vi "TwoBallAuto2safeHangar.vi"() -> ()   [LabVIEW 2020]
uses:
  Global Variables/AutoOneBall.ctl
  <vilib>/Rock Robotics/WPI/ThirdParty/REV Robotics/REVLib/Typedef/Spark MAX Control Type.ctl
  Global Variables/ActuatorsSensors.vi
  Global Variables/Axes_N_Buttons.vi
panel:
  in  "Tab Control":T1(tab)
  out "R Output":cluster{"Applied Output":dbl}(graph)
  out "L Output":cluster{"Applied Output":dbl}(graph)
  out "PID R":cluster{"Sensor Position":dbl, "Setpoint":dbl}(graph)
  out "PID L":cluster{"Sensor Position":dbl, "Setpoint":dbl}(graph)
  in  "Reset":bool
  in  "PID Constants L":T2={"P Gain"=0.007, "I Gain"=0.0002, "D Gain"=0.0, "F Gain"=0.0, "I Zone"=1000.0, "Min Output"=-1.0, "Max Output"=1.0}
  in  "PID Constants R":T2={"P Gain"=0.003, "I Gain"=0.0002, "D Gain"=0.0, "F Gain"=0.0, "I Zone"=1000.0, "Min Output"=-0.1, "Max Output"=0.1}
  in  "Range":cluster{"output high":dbl, "output low":dbl}={"output high"=0.6, "output low"=-0.6} {"output low" format="%.2f"; "output high" format="%.2f"}
  in  "Gains":T3={"proportional gain (Kc)"=0.04, "integral time (Ti, min)"=0.0, "derivative time (Td, min)"=0.0} {"derivative time (Td, min)" format="%.3f"; "integral time (Ti, min)" format="%.3f"; "proportional gain (Kc)" format="%.3f"}
  in  "Soft start":dbl=1.8 format="%#_13g"
  in  "Meters":dbl=-2.5
  in  "Meters 2":dbl=2.3
  in  "Range 2":cluster{"output high":dbl, "output low":dbl}={"output high"=0.45, "output low"=-0.45} {"output low" format="%.2f"; "output high" format="%.2f"}
  in  "Meters 3":dbl=-0.6
  in  "Meters 4":dbl=-0.6
  in  "Meters 5":dbl=-1.5
  in  "Meters 6":dbl=-1.0
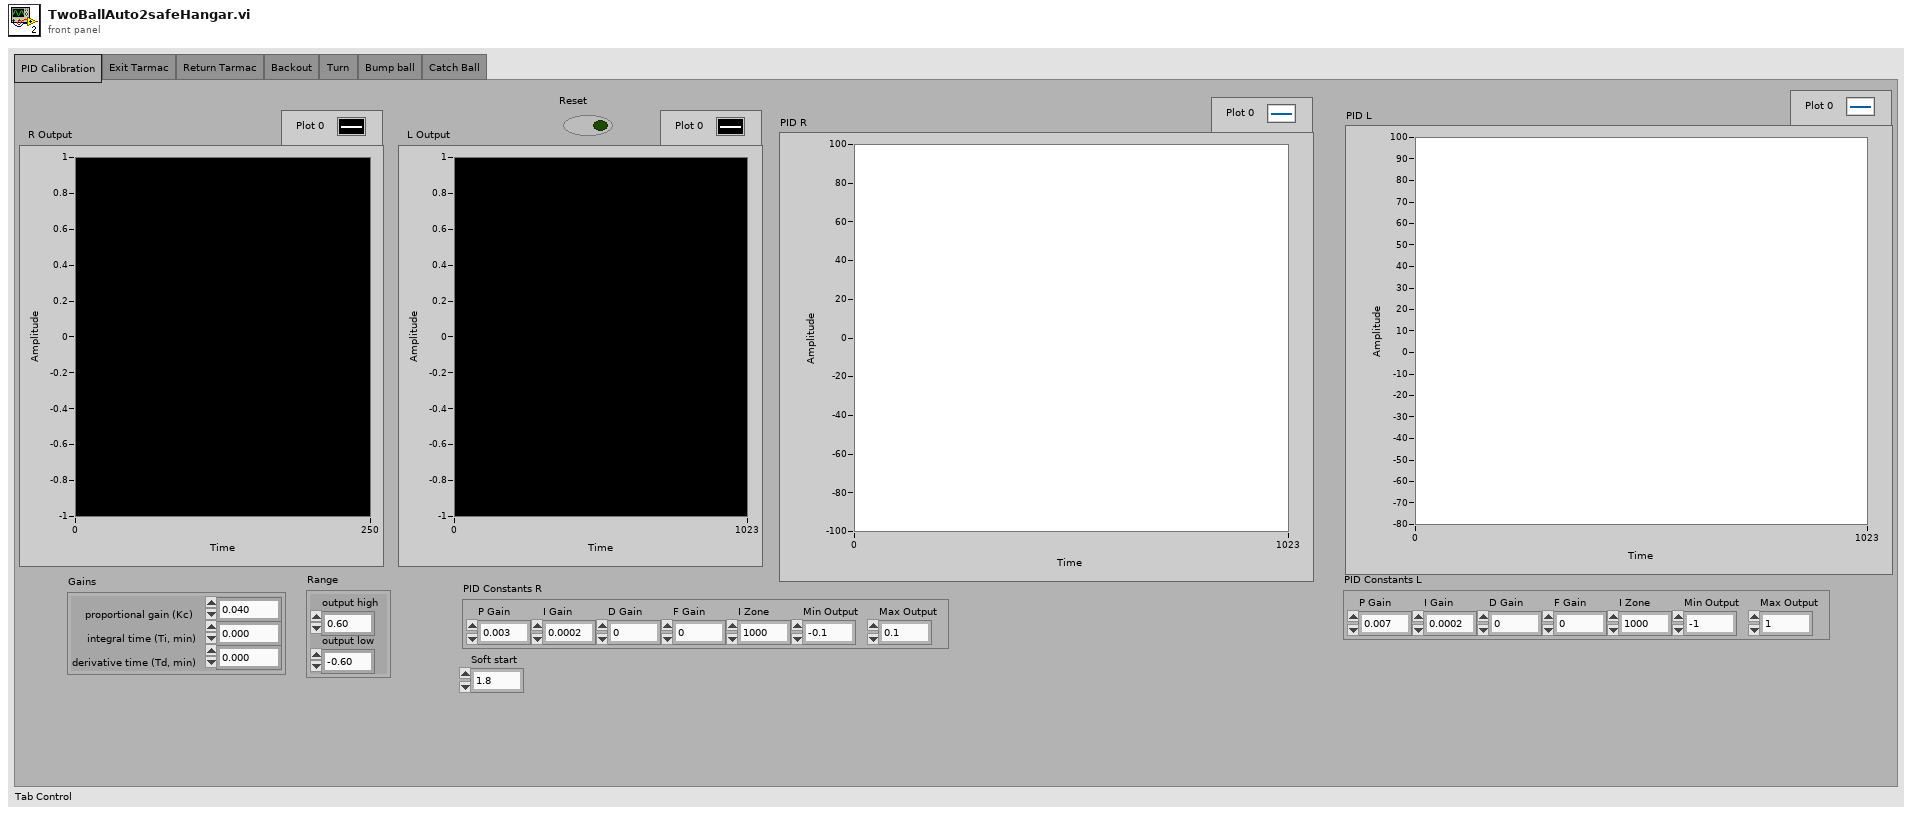
[diagram p1: front panel]
types:
  T1 = enum32{"PID Calibration", "Exit Tarmac", "Return Tarmac", "Backout", "Turn ", "Bump ball", "Catch Ball"}
  T2 = cluster{"P Gain":dbl, "I Gain":dbl, "D Gain":dbl, "F Gain":dbl, "I Zone":dbl, "Min Output":dbl, "Max Output":dbl}
  T3 = cluster{"proportional gain (Kc)":dbl, "integral time (Ti, min)":dbl, "derivative time (Td, min)":dbl}
  T4 = typedef "AutoOneBall.ctl" = enum16{"Start", "Shoot", "Delay", "Exit Tarmac", "Delay 2", "Return Tarmac", "Delay 3", "Prepare Shooter 2", "Align", "Shoot 2", "Backout", "Delay 4", "Turn", "Delay 5", "Bump Ball", "Collect Ball", "Reset"}
  T5 = typedef "WPI_MotorControlDeviceRef.ctl" = cluster{"DeviceStatus":errorcluster, "Type":T6, "PWM":cluster{"PWM Channel":T7, "DeadBand":T8}, "CAN":cluster{"Device Number":u8, "SetOutput VI Ref":variant, "GetOutput VI Ref":variant, "Enable VI Ref":variant, "Disable VI Ref":variant, "Data":variant}, "Invert":bool, "DIO PWM":cluster{"PWM \"Enable\" Channel":T7, "DIOChannel":T9, "PWM Rate":dbl}}
  T6 = typedef "WPI_MotorControlType.ctl" = enum16{"PWM", "CAN", "DIO PWM"}
  T7 = typedef "FPGA_DIOPWMChannel.ctl" = enum8{"PWM 0", "PWM 1", "PWM 2", "PWM 3", "PWM 4", "PWM 5", "PWM 6", "PWM 7", "PWM 8", "PWM 9", "PWM MXP 0", "PWM MXP 1", "PWM MXP 2", "PWM MXP 3", "PWM MXP 4", "PWM MXP 5", "PWM MXP 6", "PWM MXP 7", "PWM MXP 8", "PWM MXP 9", "Invalid"}
  T8 = typedef "WPI_PWMDeadband.ctl" = cluster{"Name":string, "maxPositivePwm":i32, "minPositivePwm":i32, "centerPwm":i32, "maxNegativePwm":i32, "minNegativePwm":i32, "angularRange":u16}
  T9 = typedef "FPGA_DIOChannel.ctl" = enum8{"DIO 0", "DIO 1", "DIO 2", "DIO 3", "DIO 4", "DIO 5", "DIO 6", "DIO 7", "DIO 8", "DIO 9", "DIO MXP 0", "DIO MXP 1", "DIO MXP 2", "DIO MXP 3", "DIO MXP 4", "DIO MXP 5", "DIO MXP 6", "DIO MXP 7", "DIO MXP 8", "DIO MXP 9", "DIO MXP 10", "DIO MXP 11", "DIO MXP 12", "DIO MXP 13", "DIO MXP 14", "DIO MXP 15", "SPI Port CS1", "SPI Port CS2", "SPI Port CS3", "SPI Port MISO", "SPI Port MOSI", "Invalid"}
  T10 = typedef "Spark MAX Control Type.ctl" = enum16{"Percent VBus", "Voltage", "Velocity", "Position", "Smart Motion", "Current", "Smart Velocity"}
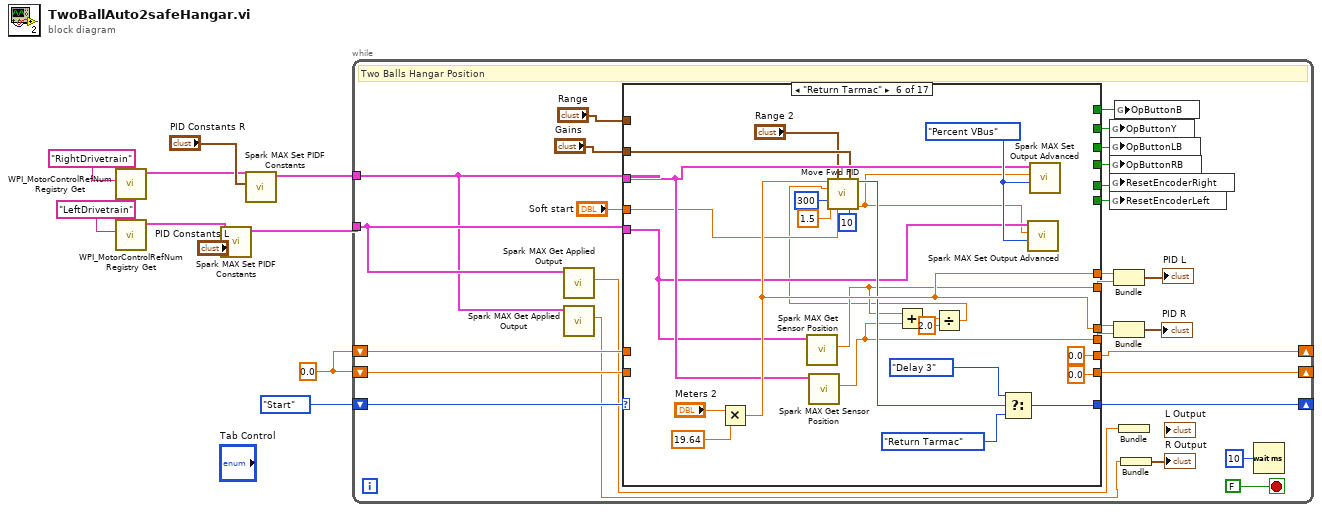
[diagram p0: block diagram]
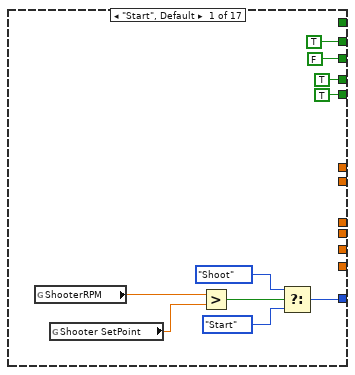
[diagram p2: hidden frame]
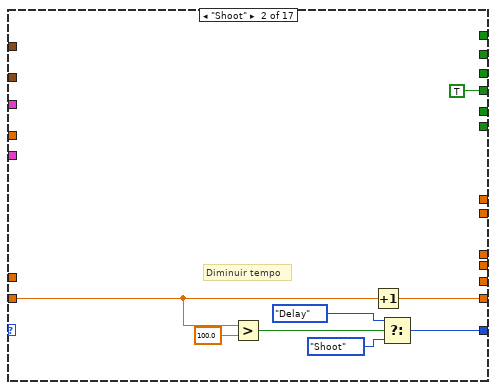
[diagram p3: hidden frame]
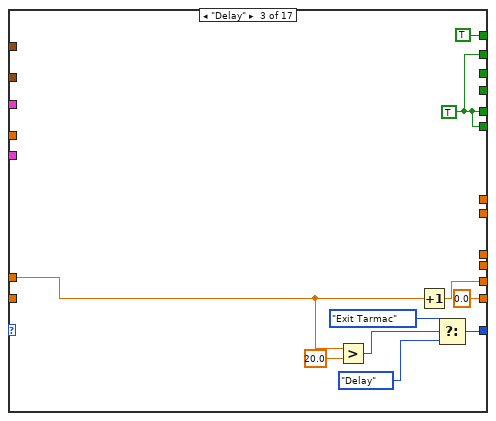
[diagram p4: hidden frame]
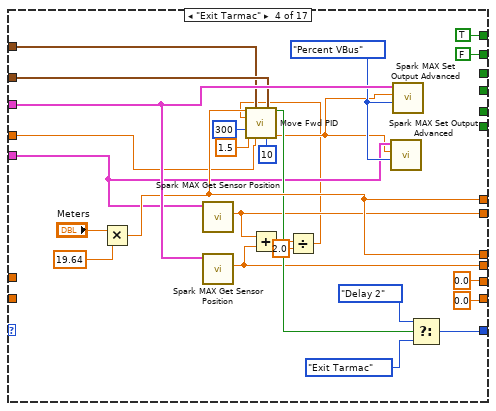
[diagram p5: hidden frame]
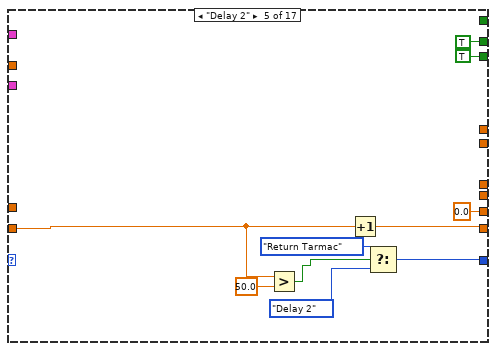
[diagram p6: hidden frame]
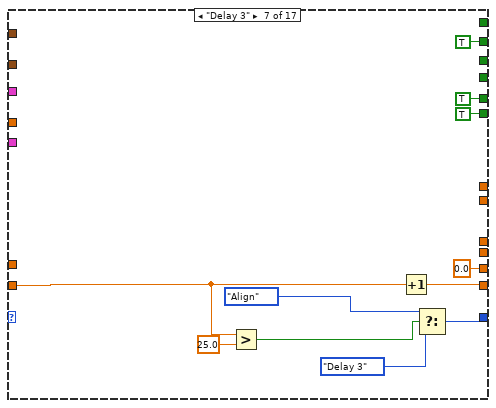
[diagram p7: hidden frame]
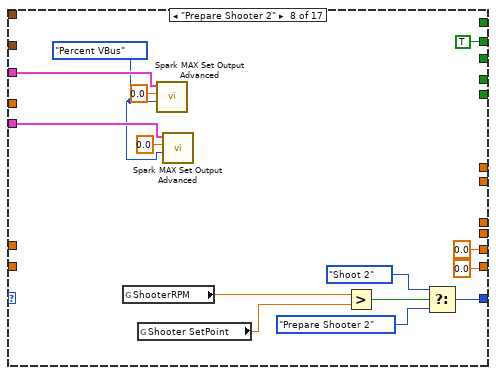
[diagram p8: hidden frame]
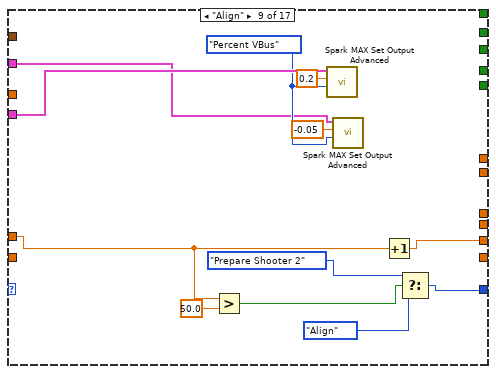
[diagram p9: hidden frame]
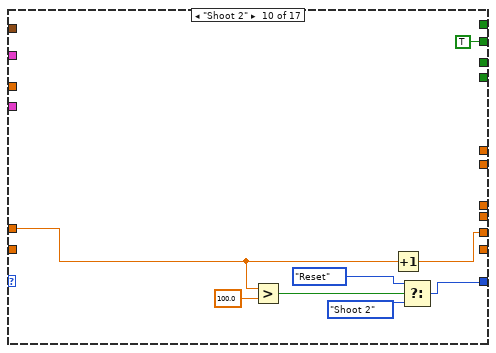
[diagram p10: hidden frame]
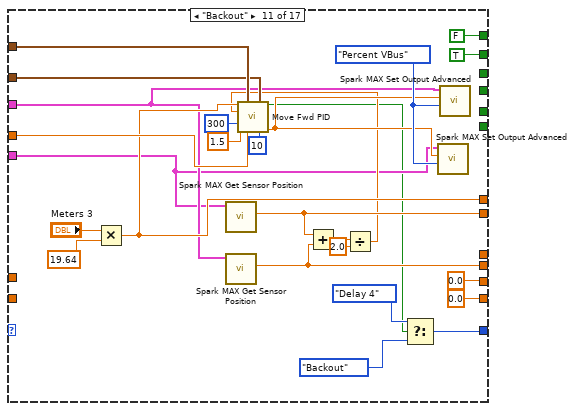
[diagram p11: hidden frame]
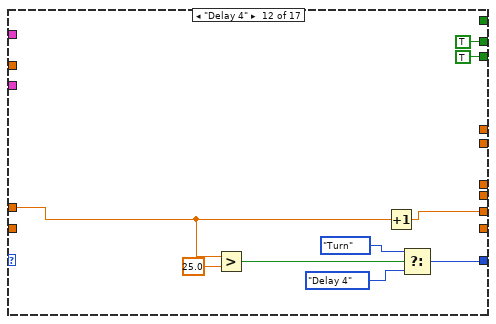
[diagram p12: hidden frame]
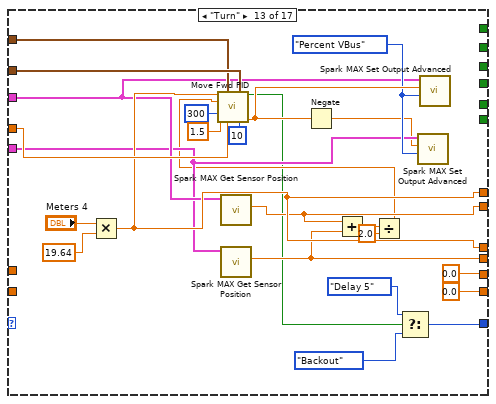
[diagram p13: hidden frame]
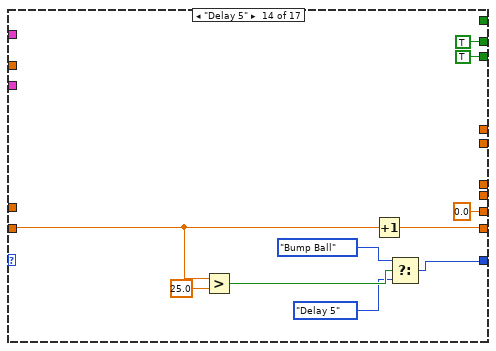
[diagram p14: hidden frame]
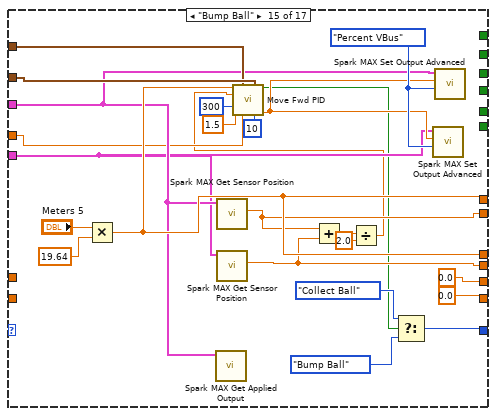
[diagram p15: hidden frame]
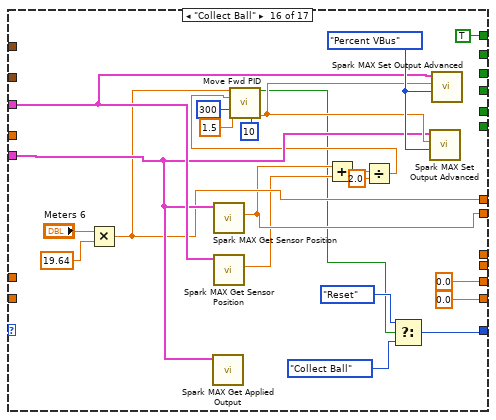
[diagram p16: hidden frame]
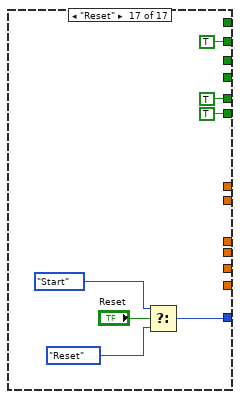
[diagram p17: hidden frame]
diagram:
  w9 = 0.0 ("Setpoint")
  n1 = call <vilib>:"WPI_MotorControlRefNum Registry Get.vi"("refnum name"="RightDrivetrain") -> ("MotorControlDevRef"=w4:T5)  [unwired: 9 in, 1 out]
  n2 = call <vilib>:"WPI_MotorControlRefNum Registry Get.vi"("refnum name"="LeftDrivetrain") -> ("MotorControlDevRef"=w3:T5)  [unwired: 9 in, 1 out]
  n3 = call <vilib>:"Spark MAX Set PIDF Constants.vi"("PID Constants"="PID Constants L", "MotorControlDeviceRef"=w3) -> ("MotorControlDeviceRef"=w2:T5)  [unwired: 8 in, 1 out]
  n4 = call <vilib>:"Spark MAX Set PIDF Constants.vi"("PID Constants"="PID Constants R", "MotorControlDeviceRef"=w4) -> ("MotorControlDeviceRef"=w1:T5)  [unwired: 8 in, 1 out]
  n5 = while {
    shift-right: [w34] -> _
    shift-left: AutoOneBall."Start" ("Enum") -> [w38]
    shift-right: [w29] -> _
    shift-left: w9 -> [w30]
    shift-right: [w20] -> _
    shift-left: w9 -> [w21]
    tunnel: w1 -> [w17]
    tunnel: w2 -> [w19]
    stop <- FALSE stop-if-true
    # "Two Balls Hangar Position"
    n6 = call <vilib>:"Spark MAX Get Applied Output.vi"("MotorControlDevRef in"=w19) -> ("Applied Output"=w13:dbl)  [unwired: 7 in, 3 out]
    n7 = call <vilib>:"Spark MAX Get Applied Output.vi"("MotorControlDevRef in"=w17) -> ("Applied Output"=w16:dbl)  [unwired: 7 in, 3 out]
    n8 = case shown="\"Return Tarmac\"" w38 {
      tunnel: w19 -> [_ _ _ w78 _ w113 _ w139 w163 _ w173 _ w214 _ w249 w273 _]
      tunnel: w17 -> [_ _ _ w84 _ w114 _ w140 w154 _ w174 _ w215 _ w250 w274 _]
      tunnel: [TRUE ("OpButtonLB") _ _ _ _ _ _ TRUE ("OpButtonLB") _ _ _ _ _ _ _ _ _] -> w35
      tunnel: [w43 w49 w65 w90 w97 w125 w130 w146 w157 w167 w191 w200 w225 w235 w261 w283 w292] -> w34
      tunnel: [_ _ _ w71 _ w106 _ _ _ _ w178 _ w212 _ w247 w269 _] -> w22
      tunnel: [_ _ _ w70 _ w107 _ _ _ _ w177 _ w211 _ w246 _ _] -> w24
      tunnel: [_ _ _ w80 _ w116 _ _ _ _ w180 _ w217 _ w253 w272 _] -> w23
      tunnel: [_ _ _ w80 _ w116 _ _ _ _ _ _ w217 _ w253 _ _] -> w25
      tunnel: [FALSE ("DrButtonRB") TRUE ("DrButtonRB") _ _ _ _ _ _ _ TRUE ("DrButtonRB") _ _ _ _ _ _ _] -> w31
      tunnel: w30 -> [_ w55 _ _ w99 _ w136 _ _ _ _ _ _ w237 _ _ _]
      tunnel: [_ w53 0.0 0.0 w98 0.0 w134 0.0 _ _ 0.0 _ 0.0 w236 0.0 0.0 _] -> w29
      tunnel: [TRUE ("ResetEncoderRight") _ w61 _ TRUE ("ResetEncoderRight") _ TRUE ("ResetEncoderRight") _ _ _ _ TRUE ("ResetEncoderRight") _ TRUE ("ResetEncoderRight") _ _ TRUE ("ResetEncoderRight")] -> w28
      tunnel: [TRUE ("ResetEncoderRight") _ w61 _ TRUE ("ResetEncoderRight") _ TRUE ("ResetEncoderRight") _ _ _ _ TRUE ("ResetEncoderRight") _ TRUE ("ResetEncoderRight") _ _ TRUE ("ResetEncoderRight")] -> w27
      tunnel: [_ _ w61 FALSE ("ResetEncoderRight") _ _ TRUE ("ResetEncoderRight") _ _ _ TRUE ("ResetEncoderRight") _ _ _ _ _ TRUE ("ResetEncoderRight")] -> w26
      tunnel: w21 -> [_ _ w60 _ _ _ _ _ w153 w165 _ w202 _ _ _ _ _]
      tunnel: [_ _ w59 0.0 0.0 0.0 0.0 0.0 w152 w164 0.0 w201 0.0 0.0 0.0 0.0 _] -> w20
      tunnel: [_ _ TRUE ("ResetEncoderRight") TRUE ("ResetEncoderRight") _ _ _ _ _ _ FALSE ("ResetEncoderRight") _ _ _ _ TRUE ("ResetEncoderRight") _] -> w18
      tunnel: "Soft start" -> [_ _ _ w75 _ w112 _ _ _ _ w181 _ w220 _ w248 _ _]
      tunnel: "Gains" -> [_ _ _ w74 _ w111 _ _ _ _ w182 _ w219 _ w252 _ _]
      tunnel: "Range" -> [_ _ _ w73 _ _ _ _ _ _ w183 _ w218 _ w251 _ _]
      frame "Start", Default {
        n9 = global read "ActuatorsSensors.vi" "ShooterRPM"() -> (w47:dbl)
        n10 = global read "ActuatorsSensors.vi" "Shooter SetPoint"() -> (w39:dbl)
        n11 = Greater?(x=w47, y=w39) -> (0:w46:bool)
        n12 = Select(t=AutoOneBall."Shoot" ("Enum"), s=w46, f=AutoOneBall."Start" ("Enum")) -> (s? t:f=w43:T4)
      }
      frame "Shoot" {
        # "Diminuir tempo"
        n13 = Greater?(x=w55, y=100.0) -> (0:w52:bool)
        n14 = Increment(x=w55) -> (x+1=w53:dbl)
        n15 = Select(t=AutoOneBall."Delay" ("Enum"), s=w52, f=AutoOneBall."Shoot" ("Enum")) -> (s? t:f=w49:T4)
      }
      frame "Delay" {
        w61 = TRUE ("ResetEncoderRight")
        n16 = Greater?(x=w60, y=20.0) -> (0:w64:bool)
        n17 = Increment(x=w60) -> (x+1=w59:dbl)
        n18 = Select(t=AutoOneBall."Exit Tarmac" ("Enum"), s=w64, f=AutoOneBall."Delay" ("Enum")) -> (s? t:f=w65:T4)
      }
      frame "Exit Tarmac" {
        w81 = Spark_MAX_Control_Type."Percent VBus" ("Control Mode")
        n19 = Multiply(x="Meters", y=19.64) -> (x*y=w80:dbl)
        n20 = call <vilib>:"Spark MAX Get Sensor Position.vi"("MotorControlDevRef in"=w78) -> ("Sensor Position"=w71:dbl)  [unwired: 7 in, 3 out]
        n21 = call <vilib>:"Spark MAX Get Sensor Position.vi"("MotorControlDevRef in"=w84) -> ("Sensor Position"=w70:dbl)  [unwired: 7 in, 3 out]
        n22 = Add(x=w71, y=w70) -> (x+y=w69:dbl)
        n23 = Divide(x=w69, y=2.0) -> (x/y=w67:dbl)
        n24 = call "Move Fwd PID.vi"("Distance"=w80, "Range"=w73, "Gains"=w74, "Encoder Count"=w67, "Time to stop"=300, "Precision"=1.5, "Soft start"=w75, "Loop Timer"=10) -> ("Finished?"=w79:bool, "Output"=w76:dbl)  [unwired: 6 in]
        n25 = call <vilib>:"Spark MAX Set Output Advanced.vi"("Control Mode"=w81, "Setpoint"=w76, "MotorControlDevRef"=w78) -> ()  [unwired: 7 in, 2 out]
        n26 = call <vilib>:"Spark MAX Set Output Advanced.vi"("Control Mode"=w81, "Setpoint"=w76, "MotorControlDevRef"=w84) -> ()  [unwired: 7 in, 2 out]
        n27 = Select(t=AutoOneBall."Delay 2" ("Enum"), s=w79, f=AutoOneBall."Exit Tarmac" ("Enum")) -> (s? t:f=w90:T4)
      }
      frame "Delay 2" {
        n28 = Greater?(x=w99, y=50.0) -> (0:w95:bool)
        n29 = Increment(x=w99) -> (x+1=w98:dbl)
        n30 = Select(t=AutoOneBall."Return Tarmac" ("Enum"), s=w95, f=AutoOneBall."Delay 2" ("Enum")) -> (s? t:f=w97:T4)
      }
      frame "Return Tarmac" {
        w117 = Spark_MAX_Control_Type."Percent VBus" ("Control Mode")
        n31 = Multiply(x="Meters 2", y=19.64) -> (x*y=w116:dbl)
        n32 = call <vilib>:"Spark MAX Get Sensor Position.vi"("MotorControlDevRef in"=w113) -> ("Sensor Position"=w106:dbl)  [unwired: 7 in, 3 out]
        n33 = call <vilib>:"Spark MAX Get Sensor Position.vi"("MotorControlDevRef in"=w114) -> ("Sensor Position"=w107:dbl)  [unwired: 7 in, 3 out]
        n34 = Add(x=w106, y=w107) -> (x+y=w105:dbl)
        n35 = Divide(x=w105, y=2.0) -> (x/y=w104:dbl)
        n36 = call "Move Fwd PID.vi"("Distance"=w116, "Range"="Range 2", "Gains"=w111, "Encoder Count"=w104, "Time to stop"=300, "Precision"=1.5, "Soft start"=w112, "Loop Timer"=10) -> ("Finished?"=w115:bool, "Output"=w109:dbl)  [unwired: 6 in]
        n37 = Select(t=AutoOneBall."Delay 3" ("Enum"), s=w115, f=AutoOneBall."Return Tarmac" ("Enum")) -> (s? t:f=w125:T4)
        n38 = call <vilib>:"Spark MAX Set Output Advanced.vi"("Control Mode"=w117, "Setpoint"=w109, "MotorControlDevRef"=w113) -> ()  [unwired: 7 in, 2 out]
        n39 = call <vilib>:"Spark MAX Set Output Advanced.vi"("Control Mode"=w117, "Setpoint"=w109, "MotorControlDevRef"=w114) -> ()  [unwired: 7 in, 2 out]
      }
      frame "Delay 3" {
        n40 = Greater?(x=w136, y=25.0) -> (0:w133:bool)
        n41 = Increment(x=w136) -> (x+1=w134:dbl)
        n42 = Select(t=AutoOneBall."Align" ("Enum"), s=w133, f=AutoOneBall."Delay 3" ("Enum")) -> (s? t:f=w130:T4)
      }
      frame "Prepare Shooter 2" {
        w138 = Spark_MAX_Control_Type."Percent VBus" ("Control Mode")
        n43 = global read "ActuatorsSensors.vi" "ShooterRPM"() -> (w149:dbl)
        n44 = global read "ActuatorsSensors.vi" "Shooter SetPoint"() -> (w151:dbl)
        n45 = call <vilib>:"Spark MAX Set Output Advanced.vi"("Control Mode"=w138, "Setpoint"=0.0, "MotorControlDevRef"=w140) -> ()  [unwired: 7 in, 2 out]
        n46 = call <vilib>:"Spark MAX Set Output Advanced.vi"("Control Mode"=w138, "Setpoint"=0.0, "MotorControlDevRef"=w139) -> ()  [unwired: 7 in, 2 out]
        n47 = Greater?(x=w149, y=w151) -> (0:w150:bool)
        n48 = Select(t=AutoOneBall."Shoot 2" ("Enum"), s=w150, f=AutoOneBall."Prepare Shooter 2" ("Enum")) -> (s? t:f=w146:T4)
      }
      frame "Align" {
        w155 = Spark_MAX_Control_Type."Percent VBus" ("Control Mode")
        n49 = Greater?(x=w153, y=50.0) -> (0:w160:bool)
        n50 = call <vilib>:"Spark MAX Set Output Advanced.vi"("Control Mode"=w155, "Setpoint"=0.2, "MotorControlDevRef"=w163) -> ()  [unwired: 7 in, 2 out]
        n51 = call <vilib>:"Spark MAX Set Output Advanced.vi"("Control Mode"=w155, "Setpoint"=-0.05, "MotorControlDevRef"=w154) -> ()  [unwired: 7 in, 2 out]
        n52 = Increment(x=w153) -> (x+1=w152:dbl)
        n53 = Select(t=AutoOneBall."Prepare Shooter 2" ("Enum"), s=w160, f=AutoOneBall."Align" ("Enum")) -> (s? t:f=w157:T4)
      }
      frame "Shoot 2" {
        n54 = Greater?(x=w165, y=100.0) -> (0:w170:bool)
        n55 = Increment(x=w165) -> (x+1=w164:dbl)
        n56 = Select(t=AutoOneBall."Reset" ("Enum"), s=w170, f=AutoOneBall."Shoot 2" ("Enum")) -> (s? t:f=w167:T4)
      }
      frame "Backout" {
        w185 = Spark_MAX_Control_Type."Percent VBus" ("Control Mode")
        n57 = Multiply(x="Meters 3", y=19.64) -> (x*y=w180:dbl)
        n58 = call <vilib>:"Spark MAX Get Sensor Position.vi"("MotorControlDevRef in"=w173) -> ("Sensor Position"=w178:dbl)  [unwired: 7 in, 3 out]
        n59 = call <vilib>:"Spark MAX Get Sensor Position.vi"("MotorControlDevRef in"=w174) -> ("Sensor Position"=w177:dbl)  [unwired: 7 in, 3 out]
        n60 = Add(x=w178, y=w177) -> (x+y=w175:dbl)
        n61 = Divide(x=w175, y=2.0) -> (x/y=w176:dbl)
        n62 = call "Move Fwd PID.vi"("Distance"=w180, "Range"=w183, "Gains"=w182, "Encoder Count"=w176, "Time to stop"=300, "Precision"=1.5, "Soft start"=w181, "Loop Timer"=10) -> ("Finished?"=w172:bool, "Output"=w184:dbl)  [unwired: 6 in]
        n63 = Select(t=AutoOneBall."Delay 4" ("Enum"), s=w172, f=AutoOneBall."Backout" ("Enum")) -> (s? t:f=w191:T4)
        n64 = call <vilib>:"Spark MAX Set Output Advanced.vi"("Control Mode"=w185, "Setpoint"=w184, "MotorControlDevRef"=w173) -> ()  [unwired: 7 in, 2 out]
        n65 = call <vilib>:"Spark MAX Set Output Advanced.vi"("Control Mode"=w185, "Setpoint"=w184, "MotorControlDevRef"=w174) -> ()  [unwired: 7 in, 2 out]
      }
      frame "Delay 4" {
        n66 = Greater?(x=w202, y=25.0) -> (0:w206:bool)
        n67 = Increment(x=w202) -> (x+1=w201:dbl)
        n68 = Select(t=AutoOneBall."Turn" ("Enum"), s=w206, f=AutoOneBall."Delay 4" ("Enum")) -> (s? t:f=w200:T4)
      }
      frame "Turn" {
        w216 = Spark_MAX_Control_Type."Percent VBus" ("Control Mode")
        n69 = Multiply(x="Meters 4", y=19.64) -> (x*y=w217:dbl)
        n70 = call <vilib>:"Spark MAX Get Sensor Position.vi"("MotorControlDevRef in"=w215) -> ("Sensor Position"=w212:dbl)  [unwired: 7 in, 3 out]
        n71 = call <vilib>:"Spark MAX Get Sensor Position.vi"("MotorControlDevRef in"=w214) -> ("Sensor Position"=w211:dbl)  [unwired: 7 in, 3 out]
        n72 = Add(x=w212, y=w211) -> (x+y=w210:dbl)
        n73 = Divide(x=w210, y=2.0) -> (x/y=w209:dbl)
        n74 = call "Move Fwd PID.vi"("Distance"=w217, "Range"=w218, "Gains"=w219, "Encoder Count"=w209, "Time to stop"=300, "Precision"=1.5, "Soft start"=w220, "Loop Timer"=10) -> ("Finished?"=w207:bool, "Output"=w221:dbl)  [unwired: 6 in]
        n75 = Negate(x=w221) -> (-x=w208:dbl)
        n76 = Select(t=AutoOneBall."Delay 5" ("Enum"), s=w207, f=AutoOneBall."Backout" ("Enum")) -> (s? t:f=w225:T4)
        n77 = call <vilib>:"Spark MAX Set Output Advanced.vi"("Control Mode"=w216, "Setpoint"=w208, "MotorControlDevRef"=w214) -> ()  [unwired: 7 in, 2 out]
        n78 = call <vilib>:"Spark MAX Set Output Advanced.vi"("Control Mode"=w216, "Setpoint"=w221, "MotorControlDevRef"=w215) -> ()  [unwired: 7 in, 2 out]
      }
      frame "Delay 5" {
        n79 = Greater?(x=w237, y=25.0) -> (0:w241:bool)
        n80 = Increment(x=w237) -> (x+1=w236:dbl)
        n81 = Select(t=AutoOneBall."Bump Ball" ("Enum"), s=w241, f=AutoOneBall."Delay 5" ("Enum")) -> (s? t:f=w235:T4)
      }
      frame "Bump Ball" {
        w255 = Spark_MAX_Control_Type."Percent VBus" ("Control Mode")
        n82 = Multiply(x="Meters 5", y=19.64) -> (x*y=w253:dbl)
        n83 = call <vilib>:"Spark MAX Get Applied Output.vi"("MotorControlDevRef in"=w250) -> ()  [unwired: 7 in, 4 out]
        n84 = call <vilib>:"Spark MAX Get Sensor Position.vi"("MotorControlDevRef in"=w250) -> ("Sensor Position"=w247:dbl)  [unwired: 7 in, 3 out]
        n85 = call <vilib>:"Spark MAX Get Sensor Position.vi"("MotorControlDevRef in"=w249) -> ("Sensor Position"=w246:dbl)  [unwired: 7 in, 3 out]
        n86 = Add(x=w247, y=w246) -> (x+y=w244:dbl)
        n87 = Divide(x=w244, y=2.0) -> (x/y=w245:dbl)
        n88 = call "Move Fwd PID.vi"("Distance"=w253, "Range"=w251, "Gains"=w252, "Encoder Count"=w245, "Time to stop"=300, "Precision"=1.5, "Soft start"=w248, "Loop Timer"=10) -> ("Finished?"=w242:bool, "Output"=w254:dbl)  [unwired: 6 in]
        n89 = Select(t=AutoOneBall."Collect Ball" ("Enum"), s=w242, f=AutoOneBall."Bump Ball" ("Enum")) -> (s? t:f=w261:T4)
        n90 = call <vilib>:"Spark MAX Set Output Advanced.vi"("Control Mode"=w255, "Setpoint"=w254, "MotorControlDevRef"=w249) -> ()  [unwired: 7 in, 2 out]
        n91 = call <vilib>:"Spark MAX Set Output Advanced.vi"("Control Mode"=w255, "Setpoint"=w254, "MotorControlDevRef"=w250) -> ()  [unwired: 7 in, 2 out]
      }
      frame "Collect Ball" {
        w276 = Spark_MAX_Control_Type."Percent VBus" ("Control Mode")
        n92 = Multiply(x="Meters 6", y=19.64) -> (x*y=w272:dbl)
        n93 = call <vilib>:"Spark MAX Get Applied Output.vi"("MotorControlDevRef in"=w273) -> ()  [unwired: 7 in, 4 out]
        n94 = call <vilib>:"Spark MAX Get Sensor Position.vi"("MotorControlDevRef in"=w273) -> ("Sensor Position"=w269:dbl)  [unwired: 7 in, 3 out]
        n95 = call <vilib>:"Spark MAX Get Sensor Position.vi"("MotorControlDevRef in"=w274) -> ("Sensor Position"=w268:dbl)  [unwired: 7 in, 3 out]
        n96 = Add(x=w269, y=w268) -> (x+y=w271:dbl)
        n97 = Divide(x=w271, y=2.0) -> (x/y=w267:dbl)
        n98 = call "Move Fwd PID.vi"("Distance"=w272, "Encoder Count"=w267, "Time to stop"=300, "Precision"=1.5, "Loop Timer"=10) -> ("Finished?"=w266:bool, "Output"=w275:dbl)  [unwired: 9 in]
        n99 = Select(t=AutoOneBall."Reset" ("Enum"), s=w266, f=AutoOneBall."Collect Ball" ("Enum")) -> (s? t:f=w283:T4)
        n100 = call <vilib>:"Spark MAX Set Output Advanced.vi"("Control Mode"=w276, "Setpoint"=w275, "MotorControlDevRef"=w273) -> ()  [unwired: 7 in, 2 out]
        n101 = call <vilib>:"Spark MAX Set Output Advanced.vi"("Control Mode"=w276, "Setpoint"=w275, "MotorControlDevRef"=w274) -> ()  [unwired: 7 in, 2 out]
      }
      frame "Reset" {
        n102 = Select(t=AutoOneBall."Start" ("Enum"), s="Reset", f=AutoOneBall."Reset" ("Enum")) -> (s? t:f=w292:T4)
      }
    }
    n103 = global write "Axes_N_Buttons.vi" "OpButtonY"(w26) -> ()
    n104 = global write "Axes_N_Buttons.vi" "OpButtonLB"(w35) -> ()
    n105 = global write "Axes_N_Buttons.vi" "OpButtonRB"(w31) -> ()
    n106 = global write "ActuatorsSensors.vi" "ResetEncoderRight"(w28) -> ()
    n107 = global write "ActuatorsSensors.vi" "ResetEncoderLeft"(w27) -> ()
    n108 = Bundle(w23, "Sensor Position"=w22) -> (→"PID L":cluster{dbl, "Sensor Position":dbl})  [unwired: 1 in]
    n109 = Bundle(w25, "Sensor Position"=w24) -> (→"PID R":cluster{dbl, "Sensor Position":dbl})  [unwired: 1 in]
    n110 = global write "Axes_N_Buttons.vi" "OpButtonB"(w18) -> ()
    n111 = Bundle("Applied Output"=w13) -> ()  [unwired: 1 in, 1 out]
    n112 = Bundle("Applied Output"=w16) -> (→"R Output":cluster{"Applied Output":dbl})  [unwired: 1 in]
    n113 = Wait (ms)(milliseconds to wait=u32 10) -> ()  [unwired: 1 out]
  }
